vi "Terminal-DriverSystem-Setter.vi"(8 "error in (no error)":errorcluster caption="错误输入（无错误）", 9 "转速":u16, 10 "启停":bool=TRUE, 11 "operation timeout (ms)":i32=5000 caption="操作超时（5000毫秒）") -> (0 "error out":errorcluster caption="错误输出")   [LabVIEW 2014]
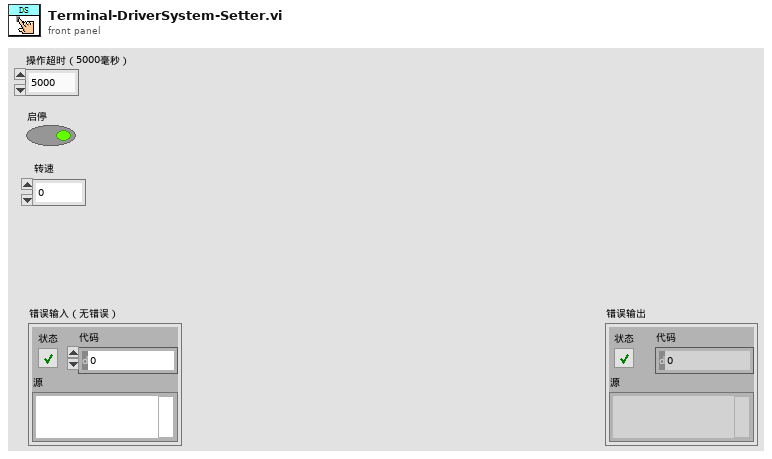
[diagram p1: front panel]
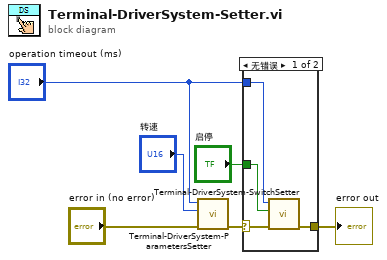
[diagram p0: block diagram]
diagram:
  n1 = call "Terminal-DriverSystem-ParametersSetter.vi"("error in (no error)"="error in (no error)", "转速"="转速", "write operation timeout (ms)"="operation timeout (ms)") -> ("error out"=w5:errorcluster)  [unwired: 8 in]
  n2 = case shown="无错误" w5 {
    selector: w5 -> [w9 w11]
    tunnel: "operation timeout (ms)" -> [w8 _]
    tunnel: [w10 w11] -> w6
    tunnel: "启停" -> [w7 _]
    frame No Error {
      n3 = call "Terminal-DriverSystem-SwitchSetter.vi"("error in (no error)"=w9, "启停"=w7, "operation timeout (ms)"=w8) -> ("error out"=w10:errorcluster)  [unwired: 8 in]
    }
    frame Error {
    }
  }
  "error out" <- w6
